vi "subDependencyInspectionCore.vi"(10 "Path to Check":path, 11 "CDependencyInspection in":refnum<class "CDependencyInspection.lvclass">) -> (3 "CDependencyInspection out":refnum<class "CDependencyInspection.lvclass">)   [LabVIEW 2020, in "DependencyInspector.lvlib"]
uses:
  DependencyInspector.lvlib
  obj/Addons/DependencyInspection.lvlibp/DependencyInspection/CDependencyInspector/CDependencyInspection.lvclass
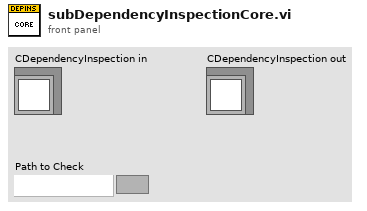
[diagram p1: front panel]
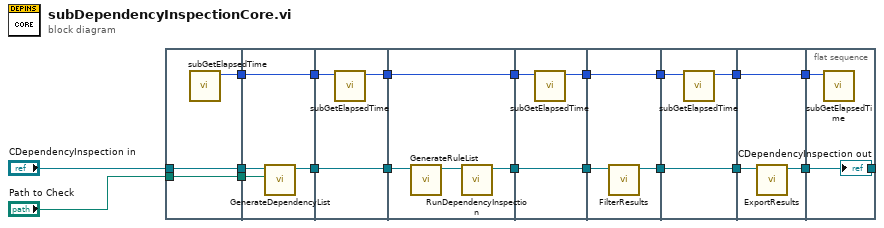
[diagram p0: block diagram]
diagram:
  n1 = flat-sequence {
    tunnel: "CDependencyInspection in" -> [w22]
    tunnel: "Path to Check" -> [w23]
    tunnel: [w23] -> w17
    tunnel: [w22] -> w16
    tunnel: [w21] -> w13
    tunnel: w17 -> [w26]
    tunnel: w16 -> [w25]
    tunnel: [w27] -> w15
    tunnel: [w24] -> w14
    tunnel: w13 -> [w24]
    tunnel: w15 -> [w30]
    tunnel: w14 -> [w29]
    tunnel: [w30] -> w12
    tunnel: [w28] -> w9
    tunnel: w12 -> [w34]
    tunnel: [w32] -> w11
    tunnel: [w31] -> w10
    tunnel: w9 -> [w31]
    tunnel: w11 -> [w37]
    tunnel: w10 -> [w36]
    tunnel: [w37] -> w6
    tunnel: [w35] -> w5
    tunnel: w6 -> [w39]
    tunnel: [w38] -> w4
    tunnel: w5 -> [w40]
    tunnel: [w40] -> w2
    tunnel: w4 -> [w43]
    tunnel: [w43] -> w3
    tunnel: w2 -> [w41]
    tunnel: [w42] -> w1
    tunnel: w3 -> [w45]
    tunnel: [w46] -> w8
    tunnel: [w44] -> w7
    tunnel: w1 -> [w44]
    tunnel: [w48] -> w20
    tunnel: w8 -> [w48]
    tunnel: w7 -> [w47]
    frame #0 {
      n2 = call "subGetElapsedTime.vi"() -> ("millisecond timer value out"=w21:u32)  [unwired: 10 in, 1 out]
    }
    frame #1 {
      n3 = call-dynamic "GenerateDependencyList.vi"("Path to Check"=w26, "CDependencyInspector in"=w25) -> ("CDependencyInspector out"=w27:refnum<class "CDependencyInspection.lvclass">)  [unwired: 6 in, 3 out]
    }
    frame #2 {
      n4 = call "subGetElapsedTime.vi"("millisecond timer value in"=w29) -> ("millisecond timer value out"=w28:u32)  [unwired: 9 in, 1 out]
    }
    frame #3 {
      n5 = call-dynamic "GenerateRuleList.vi"("CDependencyInspector in"=w34) -> ("CDependencyInspector out"=w33:refnum<class "CDependencyInspection.lvclass">)  [unwired: 9 in, 1 out]
      n6 = call-dynamic "RunDependencyInspection.vi"("CDependencyInspector in"=w33) -> ("CDependencyInspector out"=w32:refnum<class "CDependencyInspection.lvclass">)  [unwired: 9 in, 1 out]
    }
    frame #4 {
      n7 = call "subGetElapsedTime.vi"("millisecond timer value in"=w36) -> ("millisecond timer value out"=w35:u32)  [unwired: 9 in, 1 out]
    }
    frame #5 {
      n8 = call-dynamic "FilterResults.vi"("CDependencyInspection in"=w39) -> ("CDependencyInspection out"=w38:refnum<class "CDependencyInspection.lvclass">)  [unwired: 9 in, 1 out]
    }
    frame #6 {
      n9 = call "subGetElapsedTime.vi"("millisecond timer value in"=w41) -> ("millisecond timer value out"=w42:u32)  [unwired: 9 in, 1 out]
    }
    frame #7 {
      n10 = call-dynamic "ExportResults.vi"("CDependencyInspector in"=w45) -> ("CDependencyInspector out"=w46:refnum<class "CDependencyInspection.lvclass">)  [unwired: 9 in, 1 out]
    }
    frame #8 {
      n11 = call "subGetElapsedTime.vi"("millisecond timer value in"=w47) -> ()  [unwired: 9 in, 2 out]
    }
  }
  "CDependencyInspection out" <- w20
